vi "Modbus Master.vi"(7 "error in":errorcluster, 8 "Unit ID":u8=1, 9 "读取写入选择":string(combo), 10 "holding register values":u16[](array[numeric]) caption="写入保持寄存器的值", 11 "starting address":u16 caption="起始地址") -> (3 "register values":u16[](array[numeric]) caption="读取寄存器的值", 5 "error out":errorcluster)   [LabVIEW 2016, in "数据传输系统.lvlib"]
uses:
  <vilib>/NI/Modbus Library/API/Modbus API.lvclass/Modbus API.ctl
  <vilib>/NI/Modbus Library/Transmission Data Unit/Transmission Data Unit.lvclass/Transmission Data Unit.ctl
  <vilib>/NI/Modbus Library/API/Master/Set Unit ID.vi
  <vilib>/NI/Modbus Library/Transmission Data Unit/Write Unit ID.vi
  <vilib>/NI/Modbus Library/API/Read Transmission Data Unit.vi
  <vilib>/NI/Modbus Library/API/Write Transmission Data Unit.vi
  <vilib>/NI/Modbus Library/API/master/Modbus Master.lvclass
  D:/Program Files (x86)/National Instruments/LabVIEW 2016/vi.lib/NI/Modbus Library/API/Modbus API.lvclass
  <vilib>/NI/Modbus Library/API/Wrapper/Create TCP Master.vi
  <vilib>/NI/Modbus Library/API/Wrapper/API Main.lvlib
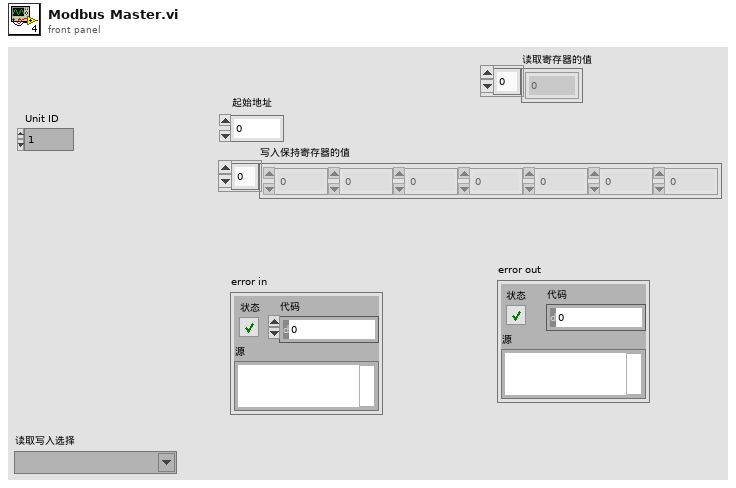
[diagram p1: front panel]
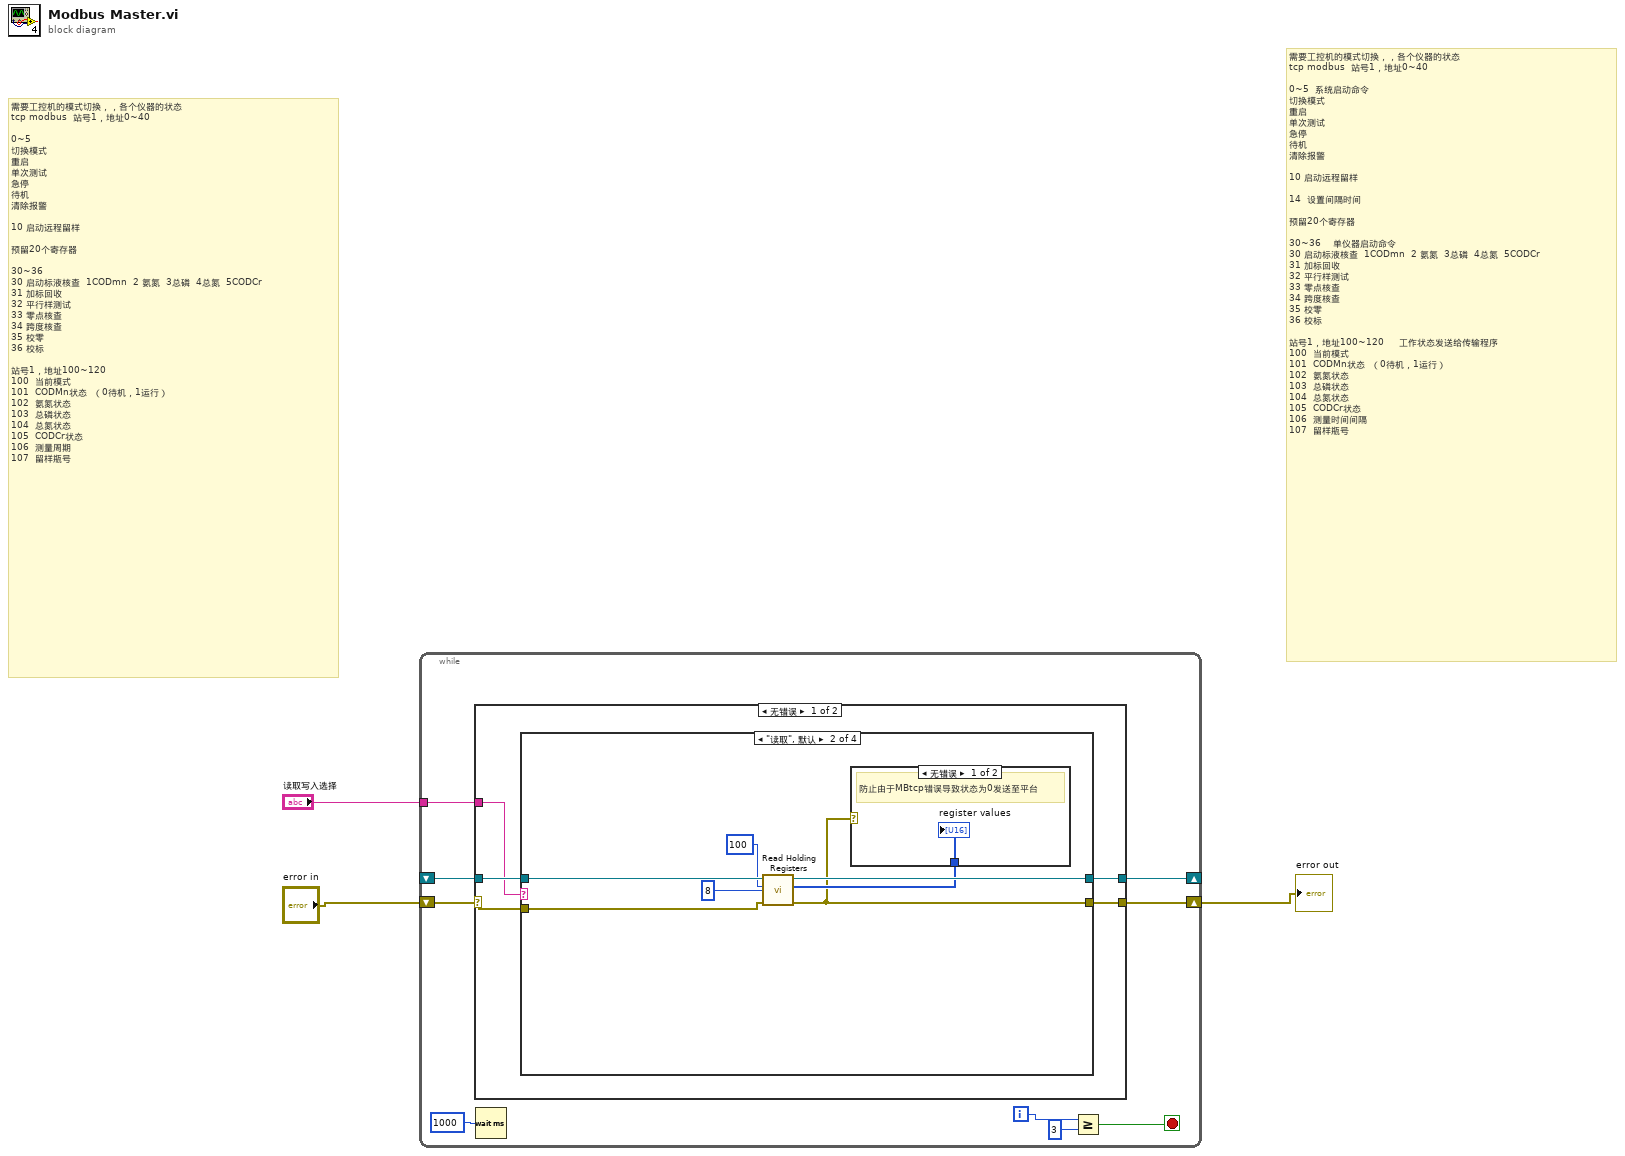
[diagram p0: block diagram]
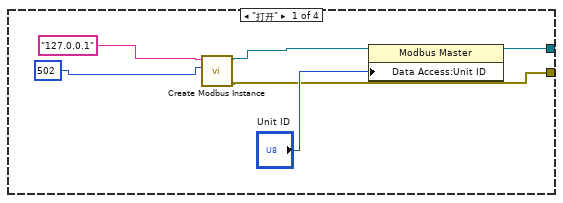
[diagram p2: hidden frame]
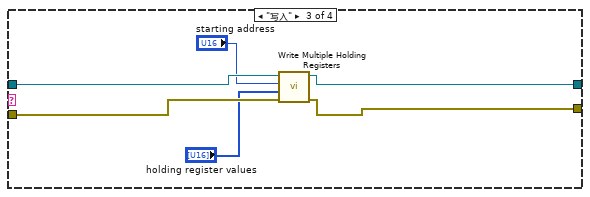
[diagram p4: hidden frame]
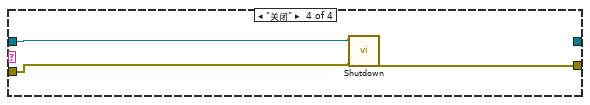
[diagram p5: hidden frame]
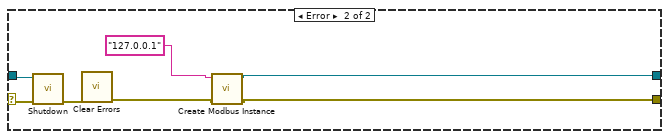
[diagram p6: hidden frame]
diagram:
  # "需要工控机的模式切换，，各个仪器的状态\ntcp modbus  站号1，地址0~40\n\n0~5  系统启动命令\n切换模式\n重启\n单次测试\n急停\n待机\n清除报警\n\n10 启动远程留样\n\n14  设置间隔时间\n\n预留20个寄存器\n\n30~36    单仪器启动命令\n30 启动标液核查  1CODmn  2 氨氮  3总磷  4总氮  5CODCr\n31 加标回收\n32 平行样测试\n33 零点核查\n34 跨度核查\n35 校零\n36 校标\n\n站号1，地址100~120     工作状态发送给传输程序\n100  当前模式\n101  CODMn状态  （0待机，1运行）\n102  氨氮状态\n103  总磷状态\n104  总氮状态\n105  CODCr状态\n106  测量时间间隔\n107  留样瓶号"
  # "需要工控机的模式切换，，各个仪器的状态\ntcp modbus  站号1，地址0~40\n\n0~5\n切换模式\n重启\n单次测试\n急停\n待机\n清除报警\n\n10 启动远程留样\n\n预留20个寄存器\n\n30~36\n30 启动标液核查  1CODmn  2 氨氮  3总磷  4总氮  5CODCr\n31 加标回收\n32 平行样测试\n33 零点核查\n34 跨度核查\n35 校零\n36 校标\n\n站号1，地址100~120\n100  当前模式\n101  CODMn状态  （0待机，1运行）\n102  氨氮状态\n103  总磷状态\n104  总氮状态\n105  CODCr状态\n106  测量周期\n107  留样瓶号"
  n1 = while {
    shift-right: [w10] -> w1
    shift-left: "error in" -> [w9]
    shift-right: [w11] -> _
    shift-left: _ -> [w12]
    tunnel: "读取写入选择" -> [w4]
    i -> [w7]
    stop <- w5 stop-if-true
    n2 = case shown="无错误" w9 {
      selector: w9 -> [w14 w41]
      tunnel: w12 -> [w17 w43]
      tunnel: [w16 w45] -> w11
      tunnel: [w15 w44] -> w10
      tunnel: w4 -> [w13 _]
      frame No Error {
        n3 = case shown="\"读取\", 默认" w13 {
          tunnel: w17 -> [_ w30 w37 w40]
          tunnel: [w20 w28 w36 _] -> w16
          tunnel: [w19 w24 w35 w38] -> w15
          tunnel: w14 -> [_ w29 w34 w39]
          frame "打开" {
            n4 = call-poly <vilib>:"Create Modbus Instance.vi"("port (502)"=u16 502, "address"="127.0.0.1") -> ("error out"=w19:errorcluster, "TCP master instance"=w23:refnum<class "Modbus Master.lvclass">)  [unwired: 8 in]
            n5 = property class="Modbus Master"(reference=w23, "Data Access:Unit ID"="Unit ID") -> (reference out=w20:refnum<class "Modbus Master.lvclass">)  [unwired: 1 in, 1 out]
          }
          frame "读取", Default {
            n6 = call-dynamic "Read Holding Registers.vi"("error in"=w29, "number of inputs"=u16 8 ("number of holding registers"), "starting address"=u16 100, "Modbus master in"=w30) -> ("error out"=w24:errorcluster, "register values"=w25:u16[], "Modbus master out"=w28:refnum<class "Modbus Master.lvclass">)  [unwired: 5 in]
            n7 = case shown="无错误" w24 {
              tunnel: w25 -> [w31 _]
              frame No Error {
                # "防止由于MBtcp错误导致状态为0发送至平台"
                "register values" <- w31
              }
              frame Error {
              }
            }
          }
          frame "写入" {
            n8 = call-dynamic "Write Multiple Holding Registers.vi"("error in"=w34, "registers to write"="holding register values", "starting address"="starting address", "Modbus master in"=w37) -> ("error out"=w35:errorcluster, "Modbus master out"=w36:refnum<class "Modbus Master.lvclass">)  [unwired: 6 in]
          }
          frame "关闭" {
            n9 = call-dynamic "Shutdown.vi"("error in"=w39, "Modbus master in"=w40) -> ("error out"=w38:errorcluster)  [unwired: 9 in]
          }
        }
      }
      frame Error {
        n10 = call-dynamic "Shutdown.vi"("error in"=w41, "Modbus master in"=w43) -> ("error out"=w42:errorcluster)  [unwired: 9 in]
        n11 = call <vilib>:"Clear Errors.vi"("error in (no error)"=w42) -> ("error out"=w46:errorcluster)  [unwired: 5 in, 1 out]
        n12 = call-poly <vilib>:"Create Modbus Instance.vi"("error in"=w46, "address"="127.0.0.1") -> ("error out"=w44:errorcluster, "TCP master instance"=w45:refnum<class "Modbus Master.lvclass">)  [unwired: 8 in]
      }
    }
    n13 = Wait (ms)(milliseconds to wait=u32 1000 ("等待时间（毫秒）")) -> ()  [unwired: 1 out]
    n14 = Greater Or Equal?(x=w7, y=3) -> (x >= y?=w5:bool)
  }
  "error out" <- w1
